vi "GetParam.vi"(8 "error in (no error)":errorcluster caption="entrée d'erreur (pas d'erreur)", 11 "ParameterGrid.lvclass":refnum<class "ParameterGrid.lvclass">) -> (0 "error out":errorcluster caption="sortie d'erreur", 2 "ParameterGrid":T1, 3 "ParameterGrid.lvclass":refnum<class "ParameterGrid.lvclass">)   [LabVIEW 2020, in "ParameterGrid.lvclass"]
doc: "Get Parameters"
uses:
  ParameterGrid.lvclass
  ParameterGrid.lvclass/ParameterGrid.ctl
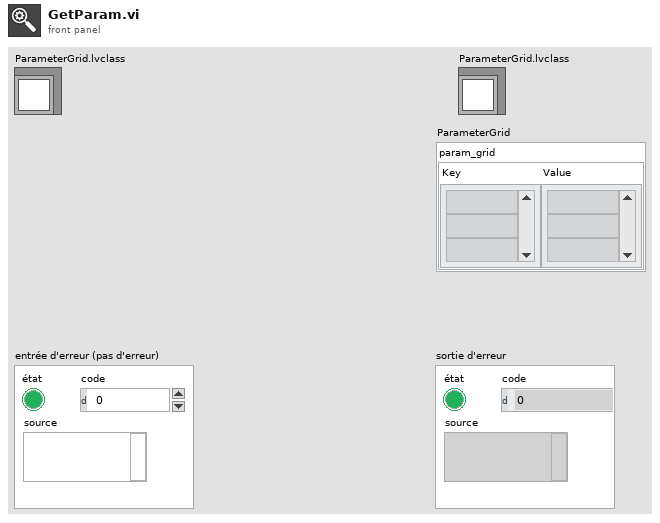
[diagram p1: front panel]
types:
  T1 = cluster{"param_grid":cluster{"Key":string[], "Value":string[]}}
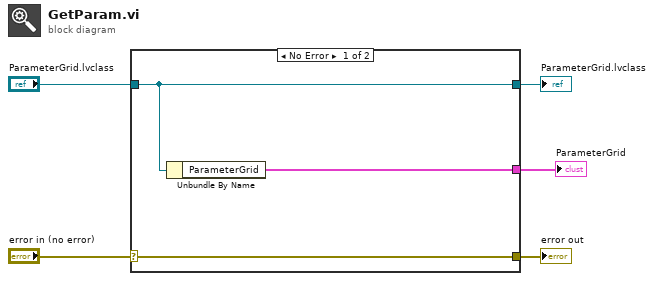
[diagram p0: block diagram]
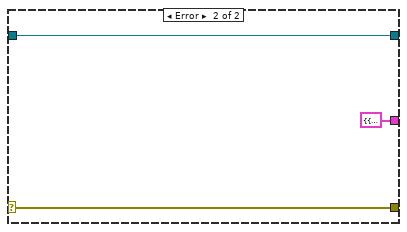
[diagram p2: hidden frame]
diagram:
  n1 = case shown="No Error" "error in (no error)" {
    selector: "error in (no error)" -> [w8 w10]
    tunnel: [w8 w10] -> w4
    tunnel: [w7 w11] -> w2
    tunnel: "ParameterGrid.lvclass" -> [w7 w11]
    tunnel: [w6 T1 {"param_grid"={"Key"=[], "Value"=[]}} ("ParameterGrid")] -> w1
    frame No Error {
      n2 = Unbundle By Name(w7) -> ("ParameterGrid"=w6:T1)
    }
    frame Error {
    }
  }
  "error out" <- w4
  "ParameterGrid.lvclass" <- w2
  "ParameterGrid" <- w1
